vi "Find Logging Section.vi"(8 "error in":errorcluster, 11 "Ballard ARINC 429 custom device in":T1 format="%.0x") -> (0 "error out":errorcluster, 2 "logging":T1 format="%.0x", 3 "Ballard ARINC 429 custom device out":T1 format="%.0x")   [LabVIEW 2020, in "Ballard ARINC 429 Scripting.lvlib"]
doc: "Within the specified <b>Ballard ARINC 429 custom device in</b>, searches for an instance of <b>port</b> with matching hardware channel number. If a match is found, returns the matching <b>port</b> reference. If no match is found, the returned reference is invalid and <b>found?</b> equals False."
uses:
  <vilib>/NI VeriStand/Custom Device API/Custom Device Item Ref.ctl
  Ballard ARINC 429 Scripting.lvlib
  <vilib>/NI VeriStand/Custom Device Tools/Custom Device Utility Library/Custom Device Utility Library.lvlib
  Constants.vi
  <vilib>/NI VeriStand/Custom Device Tools/Custom Device Utility Library/NI VeriStand - Search for Item by GUID.vi
  <vilib>/NI VeriStand/Custom Device API/Custom Device API.lvlib
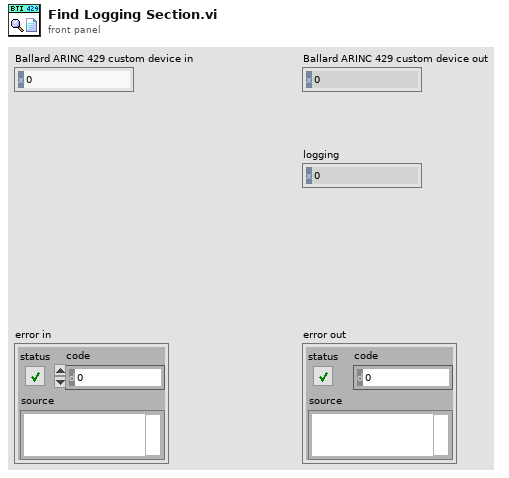
[diagram p1: front panel]
types:
  T1 = typedef "Custom Device API.lvlib/Custom Device Item Ref.ctl" = u64
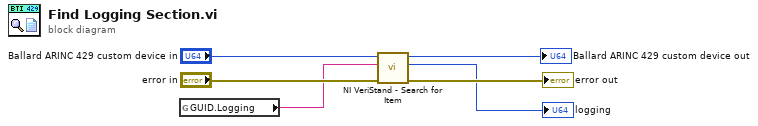
[diagram p0: block diagram]
diagram:
  n1 = global read "Constants.vi" "GUID.Logging"() -> (w4:string)
  n2 = call-poly <vilib>:"NI VeriStand - Search for Item.vi"("error in"="error in", "Item GUID"=w4, "Section Ref in"="Ballard ARINC 429 custom device in") -> ("error out"=→"error out":errorcluster, "Item Ref"=→"logging":T1, "Section Ref out"=→"Ballard ARINC 429 custom device out":T1)  [unwired: 5 in, 1 out]
